vi "GET_PRESTATUS.vi"(10 "CODE_ID":string, 11 "PRODUCT_ID":string) -> (3 "OK?":bool)   [LabVIEW 2020]
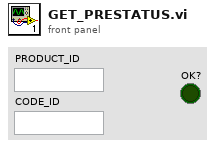
[diagram p1: front panel]
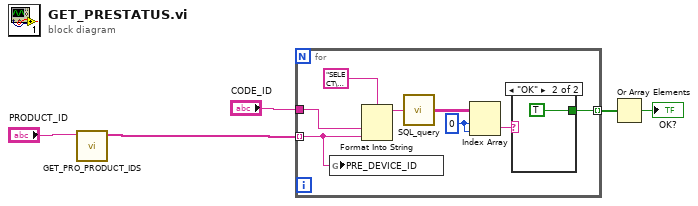
[diagram p0: block diagram]
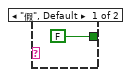
[diagram p2: hidden frame]
diagram:
  n1 = call "GET_PRO_PRODUCT_IDS.vi"("PRODUCT_ID"="PRODUCT_ID") -> ("前序工位"=w4:string[])  [unwired: 10 in]
  n2 = for {
    tunnel: w4 -> [w6] mode=indexing
    tunnel: "CODE_ID" -> [w12]
    tunnel: [w7] -> w2 mode=indexing
    w8 = 0 ("索引 (行)")
    n3 = global write "追溯Global.vi" "PRE_DEVICE_ID"(w6) -> ()
    n4 = Format Into String(format string="SELECT\ndbo.Result.RESULT_VALUE\n\nFROM\ndbo.Result\nWHERE\ndbo.Result.CODE_ID = %s AND\ndbo.Result.DEVICE_ID = %s\n" ("格式字符串"), w12, w6) -> (resulting string=w11:string)  [unwired: 2 in, 1 out]
    n5 = call "SQL_query.vi"("SQL query"=w11) -> ("data"=w10:string[][])  [unwired: 3 in, 1 out]
    n6 = Index Array(array=w10, index (row)=w8, index (col)=w8) -> (element=w9:string)
    n7 = case shown="\"OK\"" w9 {
      tunnel: [FALSE TRUE] -> w7
      frame "假", Default {
      }
      frame "OK" {
      }
    }
  }
  n8 = Or Array Elements(Boolean array=w2) -> (logical OR=→"OK?":bool)
